vi "Picture to 2-D Color Array.vi"(8 "错误输入":errorcluster, 10 "输入簇":cluster{"宽度":u32, "高度":u32}, 11 "图片":picture) -> (0 "错误输出":errorcluster, 3 "颜色数组":cluster{"红色":u8, "绿色":u8, "蓝色":u8}[][](array[cluster]))   [LabVIEW 2012]
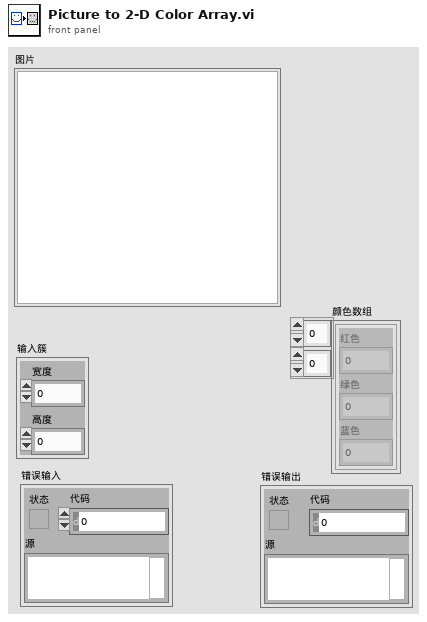
[diagram p1: front panel]
types:
  T1 = typedef "imagedata.ctl" = cluster{"image type":i32, "image depth":i32, "image":u8[], "mask":u8[], "colors":u32[], "Rectangle":cluster{"left":i16, "top":i16, "right":i16, "bottom":i16}}
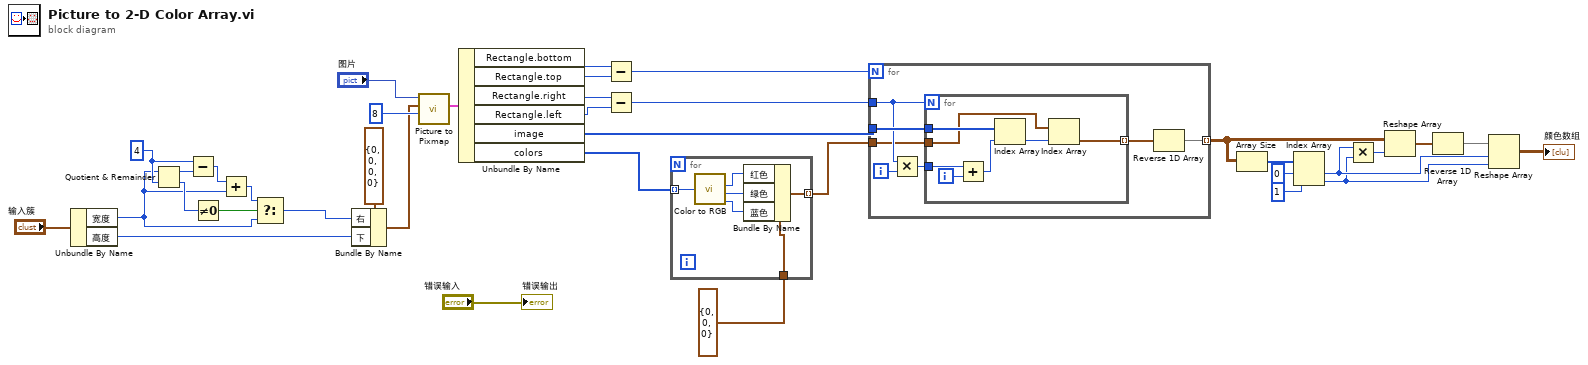
[diagram p0: block diagram]
diagram:
  w21 = 4
  n1 = Unbundle By Name ("按名称解除捆绑")("输入簇") -> ("宽度"=w4:u32, "高度"=w25:u32)
  n2 = Quotient & Remainder ("商与余数")(x=w4, y=w21) -> (x-y*floor(x/y)=w20:u32, floor(x/y)=w19:u32)
  n3 = Subtract ("减")(x=w21, y=w20) -> (x-y=w3:u32)
  n4 = Not Equal To 0? ("不等于0？")(x=w19) -> (x != 0?=w18:bool)
  n5 = Add ("加")(x=w3, y=w4) -> (x+y=w2:u32)
  n6 = Select ("选择")(t=w2, s=w18, f=w4) -> (s? t:f=w1:u32)
  n7 = Bundle By Name ("按名称捆绑")(cluster=cluster{"左":i16, "上":i16, "右":i16, "下":i16} {"左"=0, "上"=0, "右"=0, "下"=0} ("矩形"), "右"=w1, "下"=w25) -> (w22:cluster{"左":i16, "上":i16, "右":i16, "下":i16})
  n8 = call <vilib>:"Picture to Pixmap.vi"("depth"=8 ("深度"), "rect"=w22, "picture"="图片") -> ("image data"=w26:T1)  [unwired: 7 in, 1 out]
  n9 = Unbundle By Name ("按名称解除捆绑")(w26) -> ("Rectangle.bottom"=w29:i16, "Rectangle.top"=w30:i16, "Rectangle.right"=w32:i16, "Rectangle.left"=w33:i16, "image"=w35:u8[], "colors"=w8:u32[])
  n10 = Subtract ("减")(x=w29, y=w30) -> (x-y=w31:i16)
  n11 = Subtract ("减")(x=w32, y=w33) -> (x-y=w34:i16)
  n12 = for {
    tunnel: w8 -> [w42] mode=indexing
    tunnel: cluster{"红色":u8, "绿色":u8, "蓝色":u8} {"红色"=0, "绿色"=0, "蓝色"=0} ("簇") -> [w41]
    tunnel: [w37] -> w6 mode=indexing
    n13 = call <vilib>:"Color to RGB.vi"("Color"=w42) -> ("R"=w39:u8, "G"=w40:u8, "B"=w38:u8)  [unwired: 1 out]
    n14 = Bundle By Name ("按名称捆绑")(cluster=w41, "红色"=w39, "绿色"=w40, "蓝色"=w38) -> (w37:cluster{"红色":u8, "绿色":u8, "蓝色":u8})
  }
  n15 = for {
    N: w31 -> [_]
    tunnel: w6 -> [w46]
    tunnel: w34 -> [w47]
    tunnel: w35 -> [w49]
    tunnel: [w43] -> w13 mode=indexing
    i -> [w48]
    n16 = Multiply ("乘")(x=w47, y=w48) -> (x*y=w45:i32)
    n17 = for {
      N: w47 -> [_]
      tunnel: w49 -> [w56]
      tunnel: w46 -> [w51]
      tunnel: w45 -> [w55]
      tunnel: [w50] -> w44 mode=indexing
      i -> [w54]
      n18 = Add ("加")(x=w55, y=w54) -> (x+y=w53:i32)
      n19 = Index Array ("索引数组")(array=w56, index=w53) -> (element=w52:u8)
      n20 = Index Array ("索引数组")(array=w51, index=w52) -> (element=w50:cluster{"红色":u8, "绿色":u8, "蓝色":u8})
    }
    n21 = Reverse 1D Array ("反转一维数组")(array=w44) -> (reversed array=w43:cluster{"红色":u8, "绿色":u8, "蓝色":u8}[])
  }
  n22 = Array Size ("数组大小")(array=w13) -> (size(s)=w17:i32[])
  n23 = Index Array ("索引数组")(array=w17, index #1=0 ("索引"), index #2=1 ("索引")) -> (element #1=w10:i32, element #2=w9:i32)
  n24 = Multiply ("乘")(x=w10, y=w9) -> (x*y=w14:i32)
  n25 = Reshape Array ("重排数组维数")(w13, w14) -> (w12:cluster{"红色":u8, "绿色":u8, "蓝色":u8}[])
  n26 = Reverse 1D Array ("反转一维数组")(array=w12) -> (reversed array=w11:cluster{"红色":u8, "绿色":u8, "蓝色":u8}[])
  n27 = Reshape Array ("重排数组维数")(w11, w10, w9) -> (→"颜色数组":cluster{"红色":u8, "绿色":u8, "蓝色":u8}[][])
  "错误输出" <- "错误输入"
